vi "RT Main.vi"() -> ()   [LabVIEW 2011]
uses:
  TypeDefs/Recipe Engine Commands.ctl
  TypeDefs/Recipe Engine States.ctl
  <vilib>/Platform/TimedLoop/XDataNode/timing_clust.ctl
  <vilib>/Platform/TimedLoop/XDataNode/nitl_modes.ctl
  <vilib>/Platform/TimedLoop/XDataNode/wakeup.ctl
  TypeDefs/Recipe Phase.ctl
  <vilib>/Platform/TimedLoop/XDataNode/loadnilvce.vi
  <vilib>/addons/control/pid/pid.llb/PID (DBL).vi
  <vilib>/Platform/TimedLoop/XDataNode/XDataNode.xnode
  <vilib>/addons/control/pid/NI_PID_pid.lvlib
  <vilib>/Platform/TimedLoop/XDataNode/XDNodeRunTimeDep.lvlib
panel:
  out "error out":errorcluster
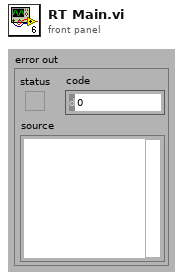
[diagram p1: front panel]
types:
  T1 = typedef "Recipe Engine Commands.ctl" = enum16{"Run Recipe", "Abort Recipe", "Exit"}
  T2 = typedef "Recipe Engine States.ctl" = enum16{"Initialize", "Wait for Cmd", "Load Phase", "Run Phase", "Exit"}
  T3 = typedef "XDNodeRunTimeDep.lvlib/timing_clust.ctl" = cluster{"Expected End [f-1]":u64, "Actual End [f-1]":u64, "Finished Late? [f-1]":bool, "Expected End [i-1]":u64, "Actual End [i-1]":u64, "Finished Late? [i-1]":bool, "Expected Start [i]":u64, "Actual Start [i]":u64, "Expected Start [f]":u64, "Actual Start [f]":u64, "Source Name":string, "Structure Name":string, "Period":i64, "Deadline":i64, "Offset":i64, "Start":i64, "Priority":i32, "Timeout":i32, "Mode":T4, "Wakeup Reason":T5, "Error":errorcluster, "Source Type":string, "Secondary Source Type":string, "Global End Time":u64, "Global Start Time":u64, "Frame Duration":u64, "Iteration Duration":u64, "Assigned CPU":i32, "I/O Scan Engine Mode":u32}
  T4 = typedef "XDNodeRunTimeDep.lvlib/nitl_modes.ctl" = enum32{"No Change", "Process missed periods, maintain original phase", "Discard missed periods, maintain original phase", "Process missed periods, ignore original phase", "Discard missed periods, ignore original phase"}
  T5 = typedef "XDNodeRunTimeDep.lvlib/wakeup.ctl" = enum32{"Normal", "Aborted", "Asynchronous wakeup", "Timing source error", "Timed loop error", "Timeout"}
  T6 = cluster{"proportional gain (Kc)":dbl, "integral time (Ti, min)":dbl, "derivative time (Td, min)":dbl}
  T7 = typedef "Recipe Phase.ctl" = cluster{"Temp Setpoint":dbl, "pH Setpoint":dbl, "Agitation ON":bool, "Intake ON":bool, "Waste ON":bool, "Time (s)":i32}
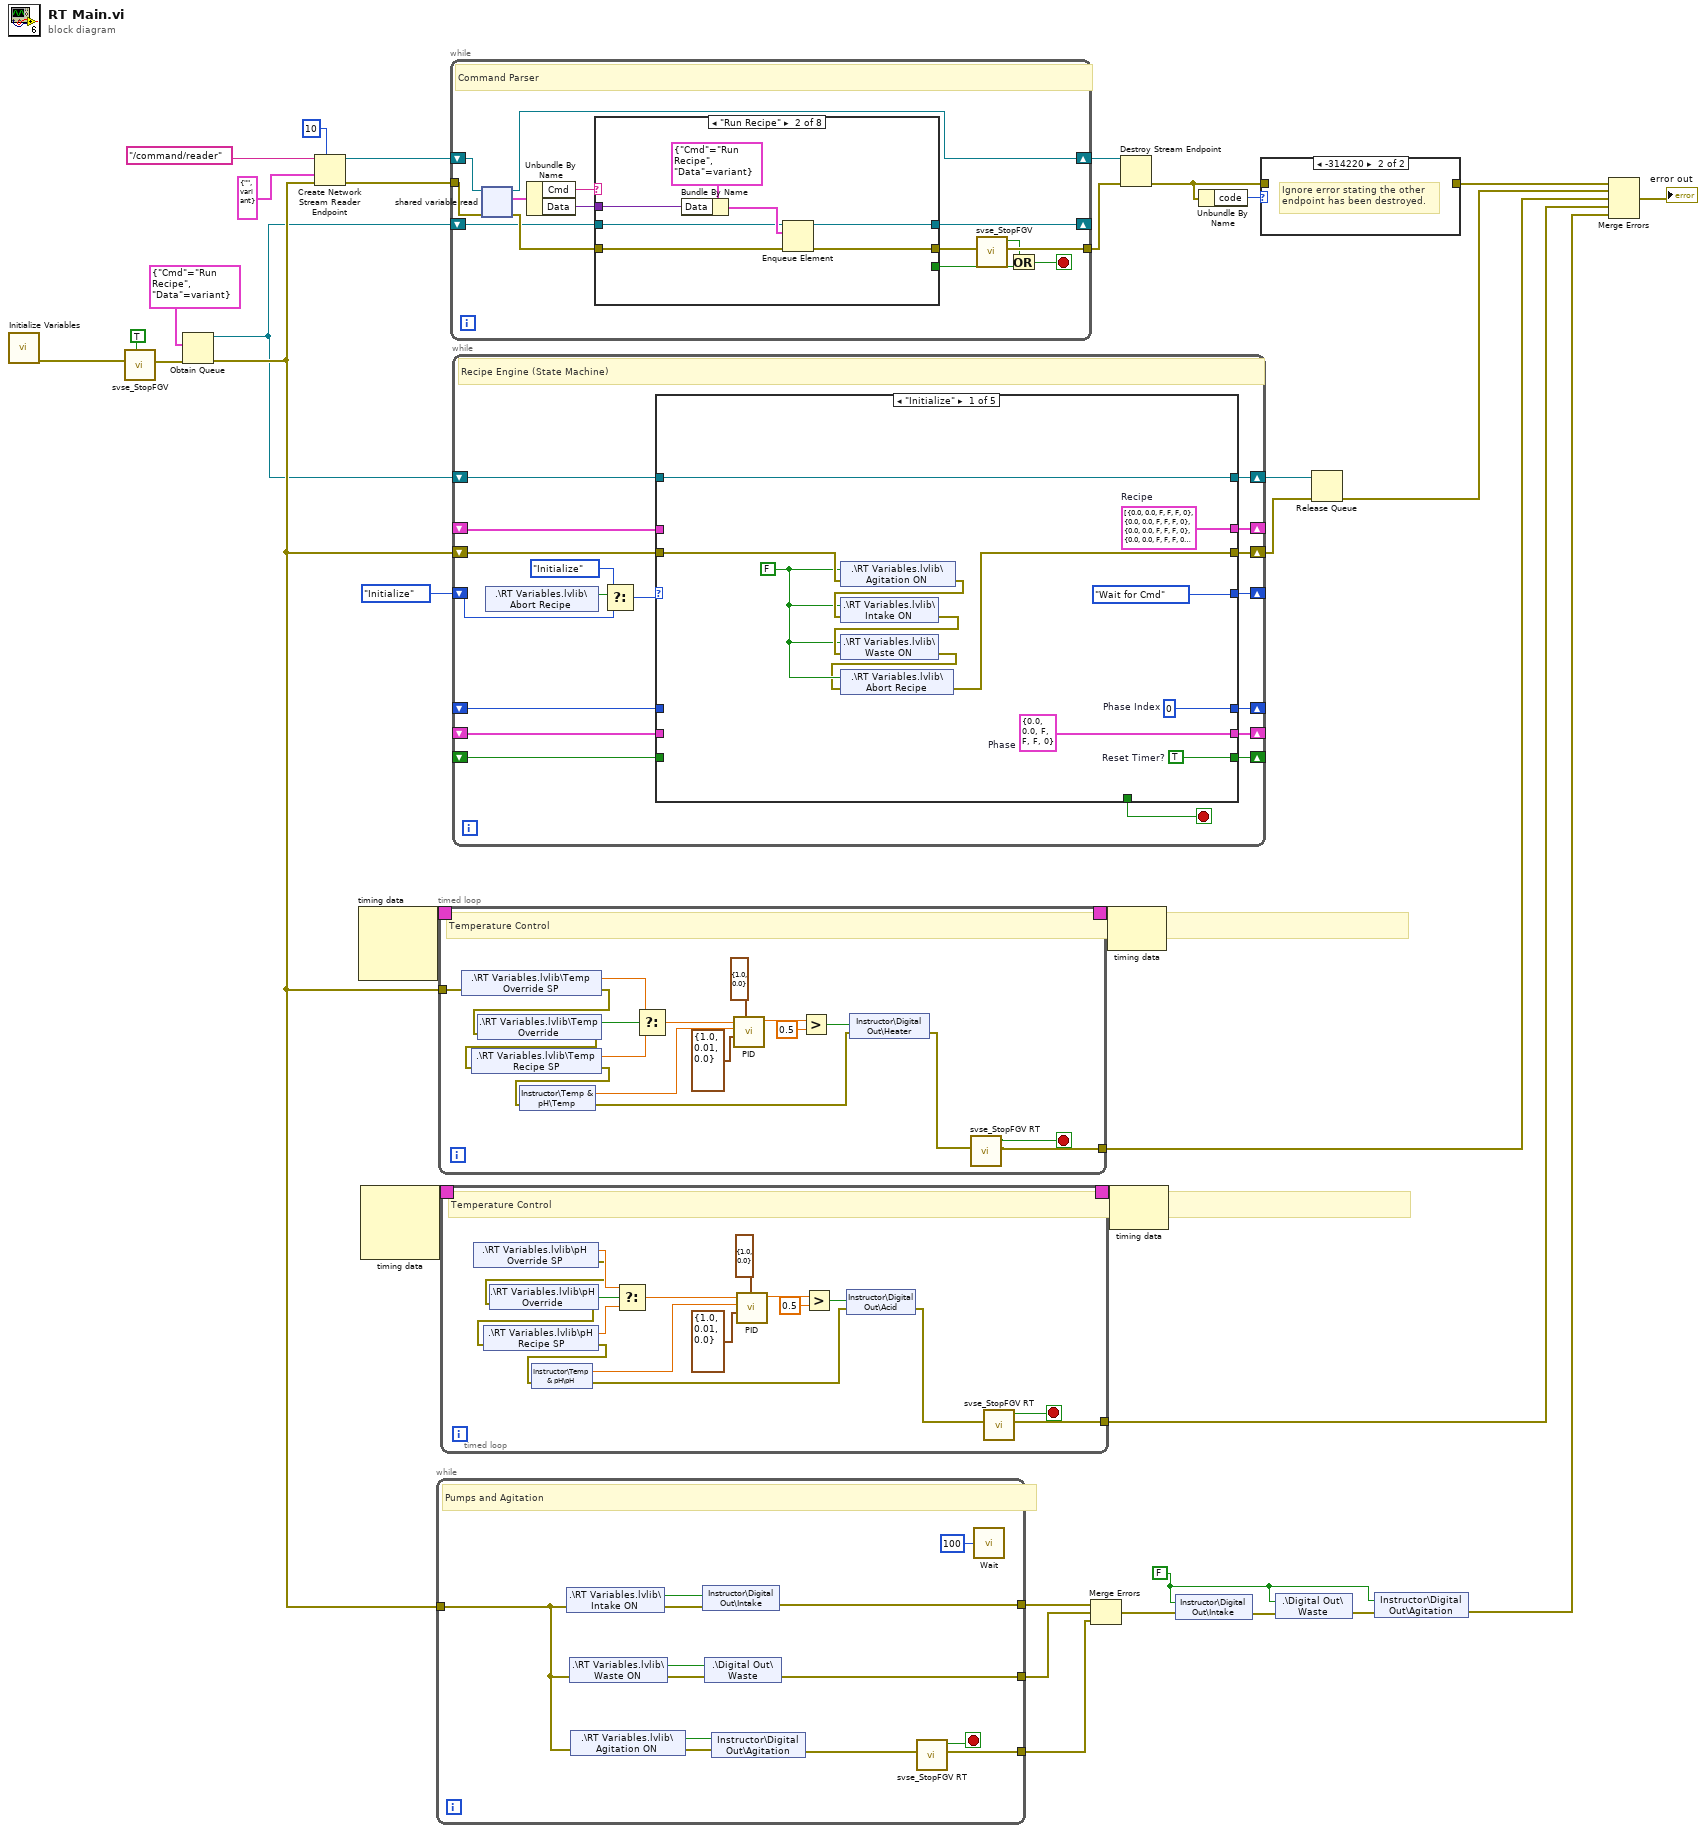
[diagram p0: block diagram]
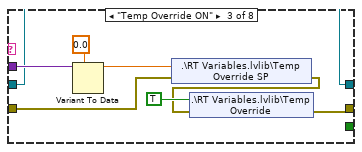
[diagram p4: hidden frame]
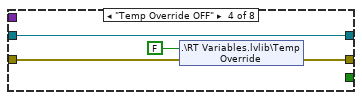
[diagram p5: hidden frame]
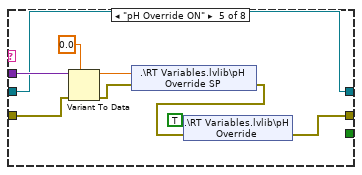
[diagram p6: hidden frame]
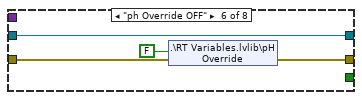
[diagram p7: hidden frame]
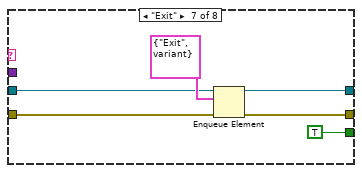
[diagram p8: hidden frame]
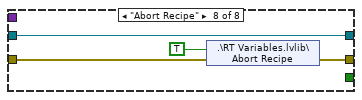
[diagram p9: hidden frame]
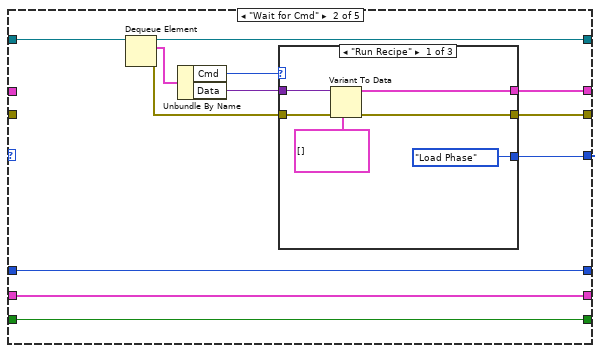
[diagram p10: hidden frame]
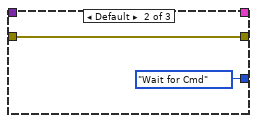
[diagram p11: hidden frame]
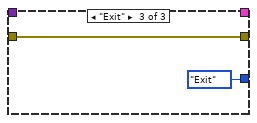
[diagram p12: hidden frame]
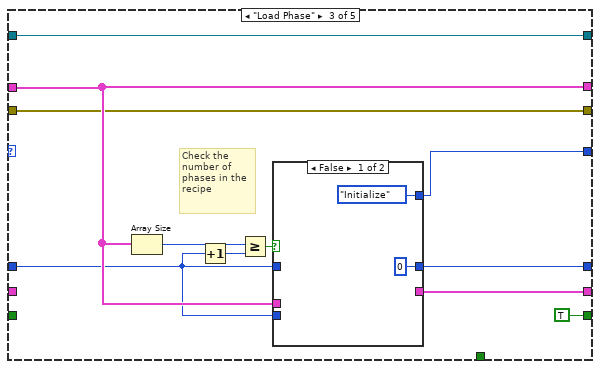
[diagram p13: hidden frame]
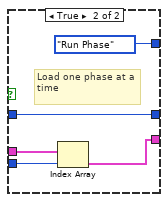
[diagram p14: hidden frame]
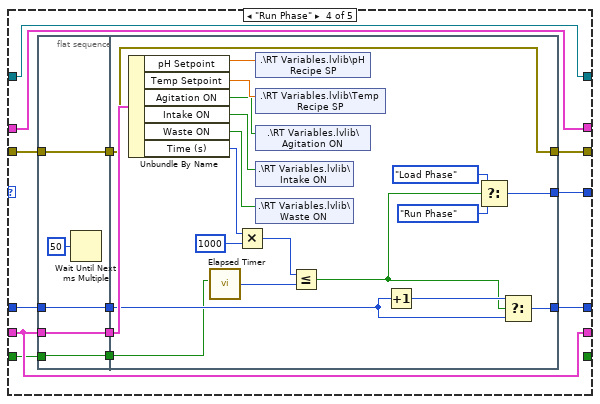
[diagram p15: hidden frame]
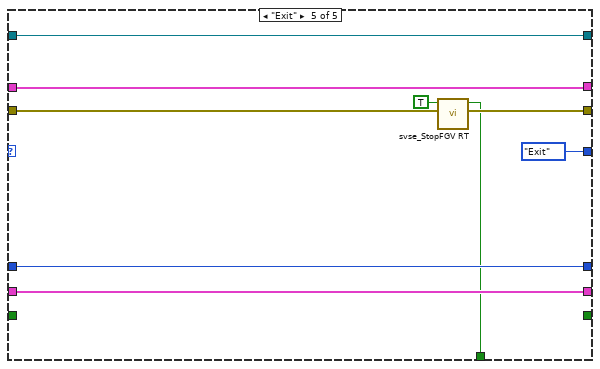
[diagram p16: hidden frame]
diagram:
  w17 = FALSE ("Intake")
  n1 = call "Initialize Variables.vi"() -> ("error out"=w11:errorcluster)  [unwired: 11 in]
  n2 = call "svse_StopFGV.vi"("Reset (F)"=TRUE, "error in"=w11) -> ("error out"=w10:errorcluster)  [unwired: 8 in, 1 out]
  n3 = Obtain Queue(element data type=cluster{"Cmd":T1, "Data":variant} {"Cmd"=enum."Run Recipe", "Data"=variant}, error in (no error)=w10) -> (queue out=w1:refnum<queue>, error out=w26:errorcluster)  [unwired: 3 in, 1 out]
  n4 = Create Network Stream Reader Endpoint(7:10 ("reader buffer size"), 8:w26, 9:cluster{"Cmd":string, "Data":variant} {"Cmd"="", "Data"=variant}, 11:"/command/reader" ("reader url")) -> (0:w29:errorcluster, 3:w31:refnum<k21>)  [unwired: 2 in]
  n5 = node-c288() -> (w28:T3)  [unwired: 3 in]
  n6 = node-c288() -> (w16:T3)  [unwired: 3 in]
  n7 = while "Temp Ctrl" {
    tunnel: w26 -> [w43]
    tunnel: [w37] -> w21
    tunnel: [w41] -> w23
    tunnel: [w40] -> w22
    stop <- w36 stop-if-true
    # "Pumps and Agitation"
    n8 = shared-variable ".\\RT Variables.lvlib\\Intake ON"(error in=w43) -> (w48:bool, error out=w45:errorcluster)
    n9 = shared-variable ".\\RT Variables.lvlib\\Waste ON"(error in=w43) -> (w47:bool, error out=w44:errorcluster)
    n10 = shared-variable ".\\RT Variables.lvlib\\Agitation ON"(error in=w43) -> (w46:bool, error out=w42:errorcluster)
    n11 = shared-variable "Instructor\\Digital Out\\Intake"(w48, error in=w45) -> (error out=w41:errorcluster)
    n12 = shared-variable ".\\Digital Out\\Waste"(w47, error in=w44) -> (error out=w40:errorcluster)
    n13 = shared-variable "Instructor\\Digital Out\\Agitation"(w46, error in=w42) -> (error out=w38:errorcluster)
    n14 = call "svse_StopFGV RT.vi"("error in"=w38) -> ("error out"=w37:errorcluster, "Stop?"=w36:bool)  [unwired: 9 in]
    n15 = call "Wait"("Count(mSec)"=u32 100) -> ()  [unwired: 1 out]
  }
  n16 = timed-loop "Temp Ctrl" {
    timing: w28 -> [_]
    timing-out: [_] -> w27
    tunnel: w26 -> [w56]
    tunnel: [w51] -> w24
    stop <- w50 stop-if-true
    # "Temperature Control"
    n17 = shared-variable ".\\RT Variables.lvlib\\Temp Override SP"(error in=w56) -> (w58:dbl, error out=w55:errorcluster)
    n18 = shared-variable ".\\RT Variables.lvlib\\Temp Override"(error in=w55) -> (w57:bool, error out=w54:errorcluster)
    n19 = shared-variable ".\\RT Variables.lvlib\\Temp Recipe SP"(error in=w54) -> (w59:dbl, error out=w53:errorcluster)
    n20 = shared-variable "Instructor\\Temp & pH\\Temp"(error in=w53) -> (w61:dbl, error out=w52:errorcluster)
    n21 = Select(t=w58, s=w57, f=w59) -> (s? t:f=w66:dbl)
    n22 = call-poly <vilib>:"PID.vi"("output range"=cluster{"output high":dbl, "output low":dbl} {"output high"=1.0, "output low"=0.0}, "PID gains"=T6 {"proportional gain (Kc)"=1.0, "integral time (Ti, min)"=0.01, "derivative time (Td, min)"=0.0}, "process variable"=w61, "setpoint"=w66) -> ("output"=w63:dbl)  [unwired: 6 in, 1 out]
    n23 = Greater?(x=w63, y=0.5) -> (0:w60:bool)
    n24 = shared-variable "Instructor\\Digital Out\\Heater"(w60, error in=w52) -> (error out=w49:errorcluster)
    n25 = call "svse_StopFGV RT.vi"("error in"=w49) -> ("error out"=w51:errorcluster, "Stop?"=w50:bool)  [unwired: 9 in]
  }
  n26 = timed-loop "Temp Ctrl" {
    timing: w16 -> [_]
    timing-out: [_] -> w15
    tunnel: [w69] -> w13
    stop <- w70 stop-if-true
    # "Temperature Control"
    n27 = shared-variable ".\\RT Variables.lvlib\\pH Override SP"() -> (w76:dbl, error out=w75:errorcluster)  [unwired: 1 in]
    n28 = shared-variable ".\\RT Variables.lvlib\\pH Override"(error in=w75) -> (w77:bool, error out=w72:errorcluster)
    n29 = shared-variable ".\\RT Variables.lvlib\\pH Recipe SP"(error in=w72) -> (w78:dbl, error out=w74:errorcluster)
    n30 = shared-variable "Instructor\\Temp & pH\\pH"(error in=w74) -> (w84:dbl, error out=w73:errorcluster)
    n31 = Select(t=w76, s=w77, f=w78) -> (s? t:f=w80:dbl)
    n32 = call-poly <vilib>:"PID.vi"("output range"=cluster{"output high":dbl, "output low":dbl} {"output high"=1.0, "output low"=0.0}, "PID gains"=T6 {"proportional gain (Kc)"=1.0, "integral time (Ti, min)"=0.01, "derivative time (Td, min)"=0.0}, "process variable"=w84, "setpoint"=w80) -> ("output"=w82:dbl)  [unwired: 6 in, 1 out]
    n33 = Greater?(x=w82, y=0.5) -> (0:w85:bool)
    n34 = shared-variable "Instructor\\Digital Out\\Acid"(w85, error in=w73) -> (error out=w71:errorcluster)
    n35 = call "svse_StopFGV RT.vi"("error in"=w71) -> ("error out"=w69:errorcluster, "Stop?"=w70:bool)  [unwired: 9 in]
  }
  n36 = while {
    shift-right: [w88] -> w4
    shift-left: w31 -> [w98]
    tunnel: w29 -> [w97]
    tunnel: [w94] -> w3
    shift-right: [w89] -> _
    shift-left: w1 -> [w90]
    stop <- w92 stop-if-true
    # "Command Parser"
    n37 = shared-variable-read(w98, w97) -> (w88:refnum<k21>, w96:errorcluster, w101:cluster{"Cmd":string, "Data":variant})  [unwired: 1 in, 1 out]
    n38 = Unbundle By Name(w101) -> ("Cmd"=w100:string, "Data"=w99:variant)
    n39 = case shown="\"Run Recipe\"" w100 {
      tunnel: w99 -> [_ w109 w118 _ w131 _ _ _]
      tunnel: w96 -> [w103 w107 w114 w121 w127 w134 w141 w144]
      tunnel: [w103 w106 w112 w120 w124 w133 w139 w143] -> w95
      tunnel: [_ _ _ _ _ _ TRUE _] -> w91
      tunnel: w90 -> [w102 w105 w111 w119 w123 w132 w137 w142]
      tunnel: [w102 w104 w111 w119 w123 w132 w136 w142] -> w89
      frame Default {
      }
      frame "Run Recipe" {
        n40 = Bundle By Name(cluster=cluster{"Cmd":T1, "Data":variant} {"Cmd"=enum."Run Recipe", "Data"=variant}, "Data"=w109) -> (w108:cluster{"Cmd":T1, "Data":variant})
        n41 = Enqueue Element(queue=w105, element=w108, error in (no error)=w107) -> (queue out=w104:refnum<queue>, error out=w106:errorcluster)  [unwired: 1 in, 1 out]
      }
      frame "Temp Override ON" {
        n42 = Variant To Data(type=0.0, Variant=w118) -> (data=w115:dbl)  [unwired: 1 in, 1 out]
        n43 = shared-variable ".\\RT Variables.lvlib\\Temp Override SP"(w115, error in=w114) -> (error out=w113:errorcluster)
        n44 = shared-variable ".\\RT Variables.lvlib\\Temp Override"(TRUE ("Temp Override"), error in=w113) -> (error out=w112:errorcluster)
      }
      frame "Temp Override OFF" {
        n45 = shared-variable ".\\RT Variables.lvlib\\Temp Override"(FALSE ("Temp Override"), error in=w121) -> (error out=w120:errorcluster)
      }
      frame "pH Override ON" {
        n46 = Variant To Data(error in=w127, type=0.0, Variant=w131) -> (data=w129:dbl, error out=w126:errorcluster)
        n47 = shared-variable ".\\RT Variables.lvlib\\pH Override SP"(w129, error in=w126) -> (error out=w125:errorcluster)
        n48 = shared-variable ".\\RT Variables.lvlib\\pH Override"(TRUE ("pH Override"), error in=w125) -> (error out=w124:errorcluster)
      }
      frame "ph Override OFF" {
        n49 = shared-variable ".\\RT Variables.lvlib\\pH Override"(FALSE ("pH Override"), error in=w134) -> (error out=w133:errorcluster)
      }
      frame "Exit" {
        n50 = Enqueue Element(queue=w137, element=cluster{"Cmd":T1, "Data":variant} {"Cmd"=enum."Exit", "Data"=variant}, error in (no error)=w141) -> (queue out=w136:refnum<queue>, error out=w139:errorcluster)  [unwired: 1 in, 1 out]
      }
      frame "Abort Recipe" {
        n51 = shared-variable ".\\RT Variables.lvlib\\Abort Recipe"(TRUE ("Abort"), error in=w144) -> (error out=w143:errorcluster)
      }
    }
    n52 = call "svse_StopFGV.vi"("error in"=w95) -> ("error out"=w94:errorcluster, "Stop?"=w93:bool)  [unwired: 9 in]
    n53 = Or(x=w93, y=w91) -> (x .or. y?=w92:bool)
  }
  n54 = while "Recipe" {
    shift-right: [w162] -> w9
    shift-left: w1 -> [w163]
    shift-right: [w161] -> _
    shift-left: _ -> [w159]
    shift-right: [w160] -> _
    shift-left: Recipe_Engine_States."Initialize" ("Enum") -> [w147]
    shift-right: [w157] -> _
    shift-left: _ -> [w158]
    shift-right: [w156] -> _
    shift-left: _ -> [w155]
    shift-right: [w154] -> _
    shift-left: _ -> [w153]
    shift-right: [w152] -> w8
    shift-left: w26 -> [w151]
    stop <- w150 stop-if-true
    # "Recipe Engine (State Machine)"
    n55 = shared-variable ".\\RT Variables.lvlib\\Abort Recipe"() -> (w149:bool)  [unwired: 1 in, 1 out]
    n56 = Select(t=Recipe_Engine_States."Initialize" ("Enum"), s=w149, f=w147) -> (s? t:f=w146:T2)
    n57 = case shown="\"Initialize\"" w146 {
      tunnel: w163 -> [w173 w187 w208 w222 w261]
      tunnel: [w173 w186 w208 w222 w261] -> w162
      tunnel: [w175 w182 w206 w221 w260] -> w161
      tunnel: [Recipe_Engine_States."Wait for Cmd" ("Enum") w181 w203 w225 Recipe_Engine_States."Exit" ("Enum")] -> w160
      tunnel: w159 -> [_ _ w206 w221 w260]
      tunnel: w158 -> [_ w177 w199 w226 w258]
      tunnel: [w170 w177 w202 w227 w258] -> w157
      tunnel: [w172 w180 w205 w228 w257] -> w156
      tunnel: w155 -> [_ w180 _ w228 w257]
      tunnel: [w171 w176 TRUE _ _] -> w154
      tunnel: w153 -> [_ w176 _ w220 _]
      tunnel: [w164 w178 w200 w216 w255] -> w152
      tunnel: w151 -> [w169 _ w200 w217 w256]
      tunnel: [_ _ _ _ w254] -> w150
      frame "Initialize" {
        w166 = FALSE ("Agitation ON")
        w170 = 0  # Phase Index
        w171 = TRUE  # Reset Timer?
        w172 = T7 {"Temp Setpoint"=0.0, "pH Setpoint"=0.0, "Agitation ON"=FALSE, "Intake ON"=FALSE, "Waste ON"=FALSE, "Time (s)"=0}  # Phase
        w175 = T7[] [{"Temp Setpoint"=0.0, "pH Setpoint"=0.0, "Agitation ON"=FALSE, "Intake ON"=FALSE, "Waste ON"=FALSE, "Time (s)"=0}, {"Temp Setpoint"=0.0, "pH Setpoint"=0.0, "Agitation ON"=FALSE, "Intake ON"=FALSE, "Waste ON"=FALSE, "Time (s)"=0}, {"Temp Setpoint"=0.0, "pH Setpoint"=0.0, "Agitation ON"=FALSE, "Intake ON"=FALSE, "Waste ON"=FALSE, "Time (s)"=0}, {"Temp Setpoint"=0.0, "pH Setpoint"=0.0, "Agitation ON"=FALSE, "Intake ON"=FALSE, "Waste ON"=FALSE, "Time (s)"=0}, {"Temp Setpoint"=0.0, "pH Setpoint"=0.0, "Agitation ON"=FALSE, "Intake ON"=FALSE, "Waste ON"=FALSE, "Time (s)"=0}, {"Temp Setpoint"=0.0, "pH Setpoint"=0.0, "Agitation ON"=FALSE, "Intake ON"=FALSE, "Waste ON"=FALSE, "Time (s)"=0}, {"Temp Setpoint"=0.0, "pH Setpoint"=0.0, "Agitation ON"=FALSE, "Intake ON"=FALSE, "Waste ON"=FALSE, "Time (s)"=0}, {"Temp Setpoint"=0.0, "pH Setpoint"=0.0, "Agitation ON"=FALSE, "Intake ON"=FALSE, "Waste ON"=FALSE, "Time (s)"=0}]  # Recipe
        n58 = shared-variable ".\\RT Variables.lvlib\\Agitation ON"(w166, error in=w169) -> (error out=w168:errorcluster)
        n59 = shared-variable ".\\RT Variables.lvlib\\Intake ON"(w166, error in=w168) -> (error out=w167:errorcluster)
        n60 = shared-variable ".\\RT Variables.lvlib\\Waste ON"(w166, error in=w167) -> (error out=w165:errorcluster)
        n61 = shared-variable ".\\RT Variables.lvlib\\Abort Recipe"(w166, error in=w165) -> (error out=w164:errorcluster)
      }
      frame "Wait for Cmd" {
        n62 = Dequeue Element(queue=w187) -> (queue out=w186:refnum<queue>, element=w185:cluster{"Cmd":T1, "Data":variant}, error out=w179:errorcluster)  [unwired: 2 in, 1 out]
        n63 = Unbundle By Name(w185) -> ("Cmd"=w184:T1, "Data"=w183:variant)
        n64 = case shown="\"Run Recipe\"" w184 {
          tunnel: w183 -> [w193 _ _]
          tunnel: [w191 _ _] -> w182
          tunnel: [Recipe_Engine_States."Load Phase" ("Enum") Recipe_Engine_States."Wait for Cmd" ("Enum") Recipe_Engine_States."Exit" ("Enum")] -> w181
          tunnel: w179 -> [w189 w194 w196]
          tunnel: [w188 w194 w196] -> w178
          frame "Run Recipe" {
            n65 = Variant To Data(error in=w189, type=T7[] [], Variant=w193) -> (data=w191:T7[], error out=w188:errorcluster)
          }
          frame Default {
          }
          frame "Exit" {
          }
        }
      }
      frame "Load Phase" {
        # "Check the number of phases in the recipe"
        n66 = Array Size(array=w206) -> (size(s)=w207:i32)
        n67 = Increment(x=w199) -> (x+1=w198:i32)
        n68 = Greater Or Equal?(x=w207, y=w198) -> (x >= y?=w204:bool)
        n69 = case shown="False" w204 {
          tunnel: w206 -> [_ w215]
          tunnel: [_ w214] -> w205
          tunnel: w199 -> [_ w213]
          tunnel: [Recipe_Engine_States."Initialize" ("Enum") Recipe_Engine_States."Run Phase" ("Enum")] -> w203
          tunnel: w199 -> [_ w211]
          tunnel: [0 ("Current Phase") w211] -> w202
          frame False {
          }
          frame True {
            # "Load one phase at a time"
            n70 = Index Array "Index Array"(array=w215, index=w213) -> (element=w214:T7)
          }
        }
      }
      frame "Run Phase" {
        n71 = flat-sequence {
          tunnel: w226 -> [w232]
          tunnel: w228 -> [w233]
          tunnel: [w233] -> w224
          tunnel: [w232] -> w223
          tunnel: w220 -> [w230]
          tunnel: [w230] -> w219
          tunnel: [w229] -> w218
          tunnel: w217 -> [w229]
          tunnel: [w251] -> w227
          tunnel: [w247] -> w225
          tunnel: w224 -> [w252]
          tunnel: w223 -> [w250]
          tunnel: w219 -> [w240]
          tunnel: w218 -> [w234]
          tunnel: [w234] -> w216
          frame #0 {
            n72 = Wait Until Next ms Multiple(millisecond multiple=u32 50) -> ()  [unwired: 1 out]
          }
          frame #1 {
            n73 = Unbundle By Name(w252) -> ("pH Setpoint"=w239:dbl, "Temp Setpoint"=w238:dbl, "Agitation ON"=w237:bool, "Intake ON"=w236:bool, "Waste ON"=w235:bool, "Time (s)"=w244:i32)
            n74 = call "Elapsed Timer.vi"("Reset Timer"=w240) -> ("Elapsed Time (ms)"=w241:u32)  [unwired: 10 in]
            n75 = Multiply(x=w244, y=1000) -> (x*y=w242:i32)
            n76 = shared-variable ".\\RT Variables.lvlib\\pH Recipe SP"(w239) -> ()  [unwired: 1 in, 1 out]
            n77 = shared-variable ".\\RT Variables.lvlib\\Temp Recipe SP"(w238) -> ()  [unwired: 1 in, 1 out]
            n78 = shared-variable ".\\RT Variables.lvlib\\Agitation ON"(w237) -> ()  [unwired: 1 in, 1 out]
            n79 = shared-variable ".\\RT Variables.lvlib\\Intake ON"(w236) -> ()  [unwired: 1 in, 1 out]
            n80 = shared-variable ".\\RT Variables.lvlib\\Waste ON"(w235) -> ()  [unwired: 1 in, 1 out]
            n81 = Less Or Equal?(x=w242, y=w241) -> (x <= y?=w245:bool)
            n82 = Increment(x=w250) -> (x+1=w249:i32)
            n83 = Select(t=Recipe_Engine_States."Load Phase" ("Enum"), s=w245, f=Recipe_Engine_States."Run Phase" ("Enum")) -> (s? t:f=w247:T2)
            n84 = Select(t=w249, s=w245, f=w250) -> (s? t:f=w251:i32)
          }
        }
      }
      frame "Exit" {
        n85 = call "svse_StopFGV RT.vi"("error in"=w256, "User stop? (F)"=TRUE) -> ("error out"=w255:errorcluster, "Stop?"=w254:bool)  [unwired: 8 in]
      }
    }
  }
  n86 = Merge Errors(w23, w22, w21) -> (w20:errorcluster)
  n87 = node-c288(w27) -> ()  [unwired: 1 out]
  n88 = node-c288(w15) -> ()  [unwired: 1 out]
  n89 = Destroy Stream Endpoint(8:w3, 11:w4) -> (0:w6:errorcluster)
  n90 = shared-variable "Instructor\\Digital Out\\Intake"(w17, error in=w20) -> (error out=w19:errorcluster)
  n91 = Unbundle By Name(w6) -> ("code"=w5:i32)
  n92 = case shown="-314220" w5 {
    tunnel: w6 -> [w262 _]
    tunnel: [w262 _] -> w2
    frame 0, Default {
    }
    frame -314220 {
      # "Ignore error stating the other\nendpoint has been destroyed."
    }
  }
  n93 = shared-variable ".\\Digital Out\\Waste"(w17, error in=w19) -> (error out=w18:errorcluster)
  n94 = Release Queue(queue=w9, error in (no error)=w8) -> (error out=w7:errorcluster)  [unwired: 1 in, 2 out]
  n95 = shared-variable "Instructor\\Digital Out\\Agitation"(w17, error in=w18) -> (error out=w14:errorcluster)
  n96 = Merge Errors(w2, w7, w24, w13, w14) -> (→"error out":errorcluster)
